vi "HandleRollerPneumatic.vi"(7 "InitState":T1=enum."Middle", 8 "error in (no error)":errorcluster, 10 "DisableOut?":bool, 11 "ButtonPressed?":bool) -> (0 "error out":errorcluster, 3 "State":T1)   [LabVIEW 2015]
doc: "If ButtonPressed? is true, switches the roller state. If DisableOut? is true, it will switch between middle and in; otherwise, it will switch in this order: in -> out -> middle -> in ..."
uses:
  DoubleSolenoidAction.ctl
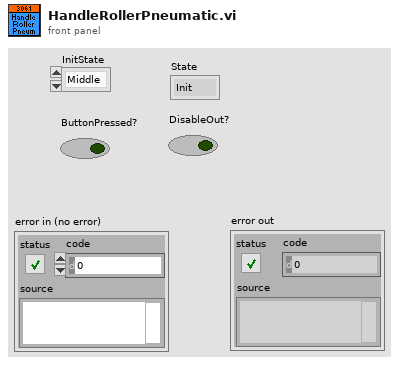
[diagram p1: front panel]
types:
  T1 = typedef "DoubleSolenoidAction.ctl" = enum16{"Init", "Middle", "In", "Out"}
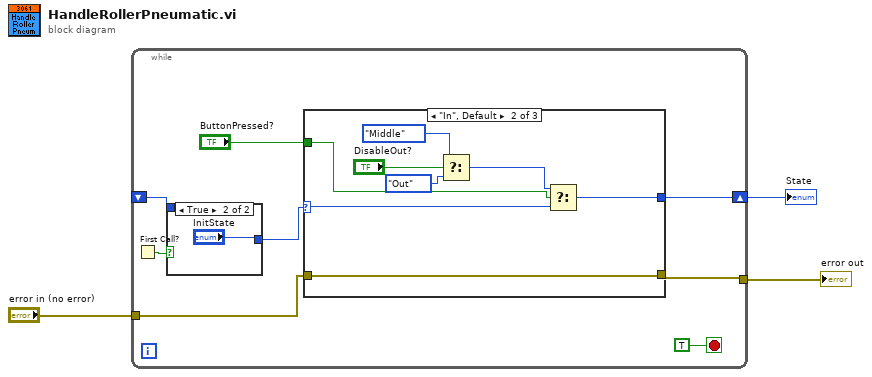
[diagram p0: block diagram]
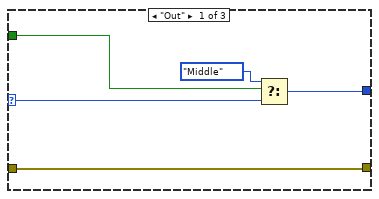
[diagram p3: hidden frame]
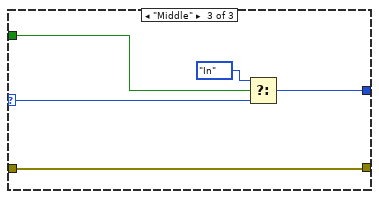
[diagram p4: hidden frame]
diagram:
  n1 = while {
    shift-right: [w10] -> w3
    shift-left: _ -> [w7]
    tunnel: "error in (no error)" -> [w5]
    tunnel: [w4] -> w1
    stop <- TRUE stop-if-true
    n2 = First Call?() -> (First Call?: T/F=w9:bool)
    n3 = case shown="True" w9 {
      tunnel: [w12 "InitState"] -> w8
      tunnel: w7 -> [w12 _]
      frame False {
      }
      frame True {
      }
    }
    n4 = case shown="\"In\", Default" w8 {
      selector: w8 -> [w16 w25 w31]
      tunnel: [w17 w26 w30] -> w10
      tunnel: "ButtonPressed?" -> [w14 w23 w27]
      tunnel: w5 -> [w15 w24 w28]
      tunnel: [w15 w24 w28] -> w4
      frame "Out" {
        n5 = Select(t=DoubleSolenoidAction."Middle", s=w14, f=w16) -> (s? t:f=w17:T1)
      }
      frame "In", Default {
        n6 = Select(t=DoubleSolenoidAction."Middle", s="DisableOut?", f=DoubleSolenoidAction."Out" ("t")) -> (s? t:f=w19:T1)
        n7 = Select(t=w19, s=w23, f=w25) -> (s? t:f=w26:T1)
      }
      frame "Middle" {
        n8 = Select(t=DoubleSolenoidAction."In", s=w27, f=w31) -> (s? t:f=w30:T1)
      }
    }
  }
  "State" <- w3
  "error out" <- w1
